vi "PH_Beckhoff_PP_PU.declare digital OutputTags.vi"(3 "PU Type":T2) -> (0 "Digital Outputs":T3, 1 "Description":string)   [LabVIEW 2014, in "PH_Beckhoff_PP_PU.lvlib"]
uses:
  PH_Beckhoff_PP_PU.lvlib
  PH_Beckhoff/PH_Beckhoff.Digital Outputs.ctl
  PH_Beckhoff_PP_PU.PU Rack Type.ctl
  PH_Beckhoff_PP_PU.Igni Tags.ctl
  PH_Beckhoff_PP_PU.RR Tags.ctl
  PH_Beckhoff/PH_Beckhoff.lvlib
panel:
  in  "Digital Input Value":T1
  out "Right Size?":bool
  # "Let this VI run to check the size!"
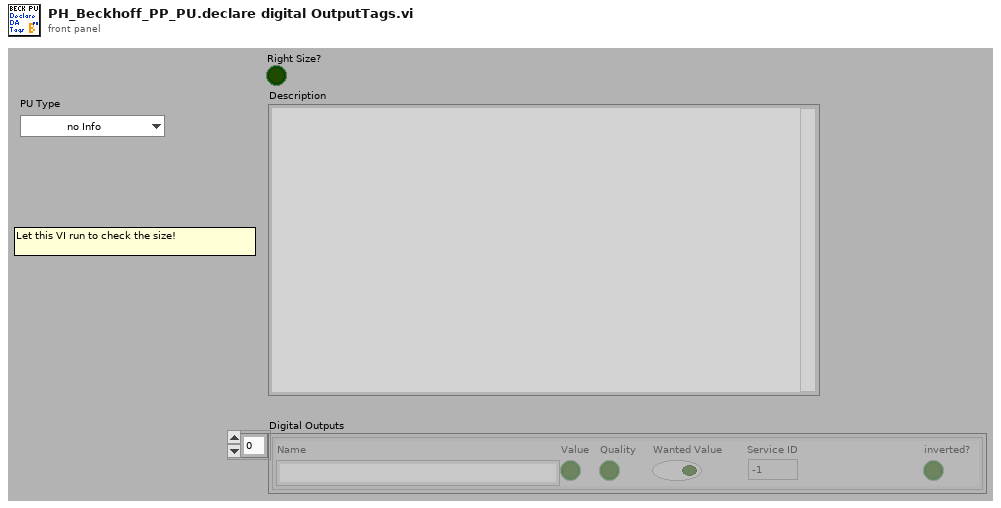
[diagram p1: front panel]
types:
  T1 = cluster{"Name":string, "Value":bool, "Quality":bool, "Wanted Value":bool, "Service ID":i32, "inverted?":bool}
  T2 = typedef "PH_Beckhoff_PP_PU.lvlib/PH_Beckhoff_PP_PU.PU Rack Type.ctl" = enum16{"no Info", "PA 19mm", "PA 45mm", "MA PU 1 and 2", "MA PU 3 and 4", "MA PU 5 and 6", "MA FR and PILC"}
  T3 = typedef "PH_Beckhoff.lvlib/PH_Beckhoff.Digital Outputs.ctl" = cluster{"Name":string, "Value":bool, "Quality":bool, "Wanted Value":bool, "Service ID":i32, "inverted?":bool}[]
  T4 = typedef "PH_Beckhoff_PP_PU.lvlib/PH_Beckhoff_PP_PU.RR Tags.ctl" = enum16{"open", "closed", "close", "Status"}
  T5 = typedef "PH_Beckhoff_PP_PU.lvlib/PH_Beckhoff_PP_PU.Igni Tags.ctl" = enum16{"heating-on", "water-on", "Device-on", "Status"}
  T6 = typedef "PH_PP_Common.lvlib/PH_PP_Common.PUs.ctl" = enum16{"no Info", "PA-19mm-1", "PA-19mm-2", "PA-45mm-PILC", "PA-45mm-MAIN", "MA-PU-1", "MA-PU-2", "MA-PU-3", "MA-PU-4", "MA-PU-5", "MA-PU-6", "MA-FR", "MA-PILC", "PA-45mm-DP"}
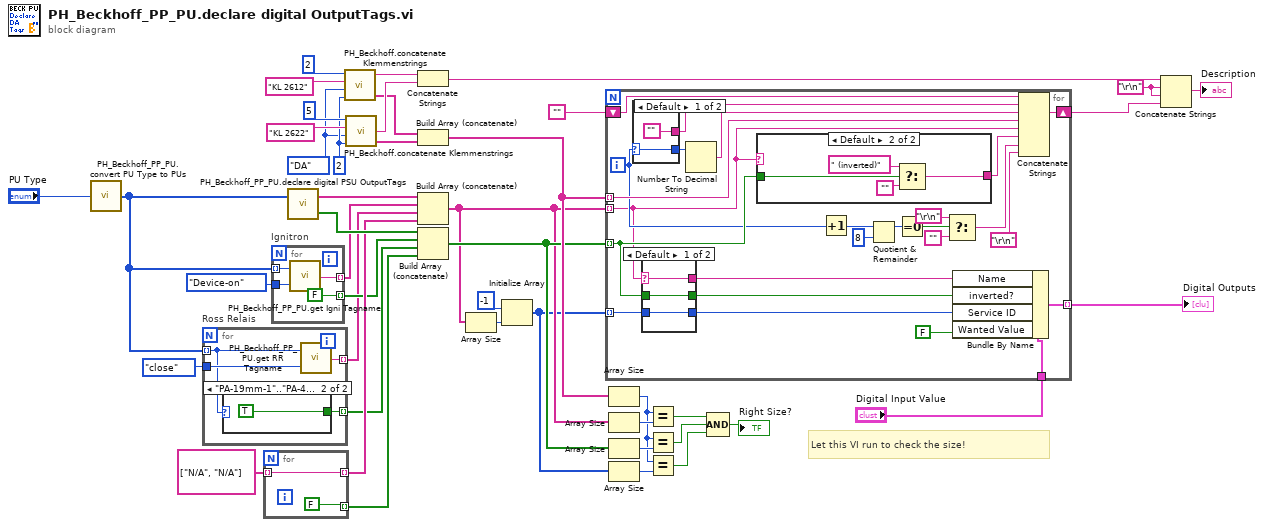
[diagram p0: block diagram]
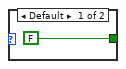
[diagram p2: hidden frame]
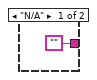
[diagram p3: hidden frame]
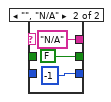
[diagram p4: hidden frame]
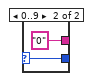
[diagram p5: hidden frame]
diagram:
  w13 = enum16{"AE", "AA", "DE", "DA", "SE"}."DA" ("Type")
  w14 = 2 ("# of In- or Outputs")
  w42 = "\r\n"
  # "Let this VI run to check the size!"
  n1 = call "PH_Beckhoff_PP_PU.convert PU Type to PUs.vi"("PU Type"="PU Type") -> ("PUs"=w6:T6[])
  n2 = for "Ross Relais" {
    tunnel: [w48] -> w7 mode=indexing
    tunnel: [w47] -> w8 mode=indexing
    tunnel: w6 -> [w45] mode=indexing
    tunnel: PH_Beckhoff_PP_PU.RR_Tags."close" ("Ross Relais Tag") -> [w46]
    n3 = case shown="\"PA-19mm-1\"..\"PA-45mm-MAIN\"" w45 {
      tunnel: [FALSE ("element") TRUE ("element")] -> w48
      frame Default {
      }
      frame "PA-19mm-1".."PA-45mm-MAIN" {
      }
    }
    n4 = call "PH_Beckhoff_PP_PU.get RR Tagname.vi"("Ross Relais Tag"=w46, "PU"=w45) -> ("RR Tagname"=w47:string)
  }
  n5 = for {
    tunnel: string[] ["N/A", "N/A"] -> [w52] mode=indexing
    tunnel: [w52] -> w19 mode=indexing
    tunnel: [FALSE ("element")] -> w18 mode=indexing
  }
  n6 = for "Ignitron" {
    tunnel: [FALSE ("element")] -> w15 mode=indexing
    tunnel: [w55] -> w16 mode=indexing
    tunnel: w6 -> [w54] mode=indexing
    tunnel: PH_Beckhoff_PP_PU.Igni_Tags."Device-on" ("Igni Tag") -> [w53]
    n7 = call "PH_Beckhoff_PP_PU.get Igni Tagname.vi"("Igni Tag"=w53, "PU"=w54) -> ("Igni Tagname"=w55:string)
  }
  n8 = call "PH_Beckhoff_PP_PU.declare digital PSU OutputTags.vi"("PUs"=w6) -> ("inverted?"=w20:bool[], "Tagnames"=w12:string[])  [unwired: 1 in]
  n9 = call "PH_Beckhoff.concatenate Klemmenstrings.vi"("# of In- or Outputs"=w14, "Type"=w13, "Klemmenname"="KL 2612", "Quantity"=2 ("size(s)")) -> ("concatenated string array"=w27:string[], "\"<Type>: <Quantity> x <Klemmenname>\""=w35:string)  [unwired: 1 out]
  n10 = call "PH_Beckhoff.concatenate Klemmenstrings.vi"("# of In- or Outputs"=w14, "Type"=w13, "Klemmenname"="KL 2622", "Quantity"=5 ("size(s)")) -> ("concatenated string array"=w28:string[], "\"and <Quantity> x <Klemmenname>\""=w36:string)  [unwired: 1 out]
  n11 = Concatenate Strings(w35, w36) -> (w34:string)
  n12 = Build Array (concatenate)(w27, w28) -> (w26:string[])
  n13 = Build Array (concatenate)(w12, w16, w8, w19) -> (w3:string[])
  n14 = Build Array (concatenate)(w20, w15, w7, w18) -> (w24:bool[])
  n15 = Array Size(array=w3) -> (size(s)=w4:i32)
  n16 = Initialize Array(-1 ("Service ID"), w4) -> (w2:i32[])
  n17 = for {
    tunnel: w3 -> [w60] mode=indexing
    tunnel: w26 -> [w69] mode=indexing
    shift-right: [w72] -> w43
    shift-left: "" -> [w73]
    tunnel: "Digital Input Value" -> [w59]
    tunnel: [w78] -> w33 mode=indexing
    tunnel: w24 -> [w74] mode=indexing
    tunnel: w2 -> [w77] mode=indexing
    i -> [w62]
    n18 = case shown="Default" w62 {
      selector: w62 -> [w93 w96]
      tunnel: [w93 w96] -> w81
      tunnel: ["" "0"] -> w80
      frame Default {
      }
      frame 0..9 {
      }
    }
    n19 = case shown="Default" w60 {
      selector: w60 -> [w87 _]
      tunnel: w77 -> [w89 _]
      tunnel: [w89 -1 ("Service ID")] -> w76
      tunnel: w74 -> [w88 _]
      tunnel: [w88 FALSE ("element")] -> w75
      tunnel: [w87 "N/A"] -> w58
      frame Default {
      }
      frame "", "N/A" {
      }
    }
    n20 = Number To Decimal String(number=w81) -> (decimal integer string=w79:string)  [unwired: 1 in]
    n21 = case shown="Default" w60 {
      tunnel: w74 -> [_ w86]
      tunnel: ["" w83] -> w71
      frame "N/A" {
      }
      frame Default {
        n22 = Select(t=" (inverted)" ("string"), s=w86, f="") -> (s? t:f=w83:string)
      }
    }
    n23 = Increment(x=w62) -> (x+1=w64:i32)
    n24 = Quotient & Remainder(x=w64, y=8) -> (x-y*floor(x/y)=w66:i32)  [unwired: 1 out]
    n25 = Equal To 0?(x=w66) -> (x = 0?=w67:bool)
    n26 = Select(t="\r\n", s=w67, f="") -> (s? t:f=w63:string)
    n27 = Bundle By Name(cluster=w59, "Name"=w58, "inverted?"=w75, "Service ID"=w76, "Wanted Value"=FALSE) -> (w78:T1)
    n28 = Concatenate Strings(w73, w80, w79, w69, w60, w71, w63, "\r\n") -> (w72:string)
  }
  "Digital Outputs" <- w33
  n29 = Array Size(array=w26) -> (size(s)=w22:i32)
  n30 = Array Size(array=w3) -> (size(s)=w25:i32)
  n31 = Array Size(array=w24) -> (size(s)=w23:i32)
  n32 = Array Size(array=w2) -> (size(s)=w32:i32)
  n33 = Equal?(x=w22, y=w25) -> (x = y?=w31:bool)
  n34 = Equal?(x=w22, y=w23) -> (x = y?=w21:bool)
  n35 = Equal?(x=w22, y=w32) -> (x = y?=w30:bool)
  n36 = Compound Arithmetic op=AND(w31, w21, w30) -> (→"Right Size?":bool)
  n37 = Concatenate Strings(w34, w42, w42, w43) -> (→"Description":string)
